vi "rqcBob Read.vi"   [LabVIEW 2019, in "rqcBob.lvclass"]
uses:
  rqcBob.lvclass
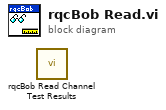
[diagram p0: block diagram]
diagram:
  n1 = call "rqcBob Read Channel Test Results.vi"() -> ()  [unwired: 13 in, 3 out]
